vi "LSCI332 GetCtrlMode.vi"(0 "VISA Rsrc":refnum<visa-resource-name>="GPIB0::12::INSTR", 5 "Boucle(1)":u32(ring) caption="Boucle" items=["Boucle 1", "Boucle 2"], 11 "error in (no error)":errorcluster) -> (4 "Mode":u32(ring)=1 items=["Manual PID"=1, "Zone"=2, "Open Loop"=3, "AutoTune PID"=4, "AutoTune PI"=5, "AutoTune P"=6], 15 "error out":errorcluster)   [LabVIEW 2019]
doc: "Ce VI lit les paramètres limites de contrôle et ceux de stabilisation du contrôleur."
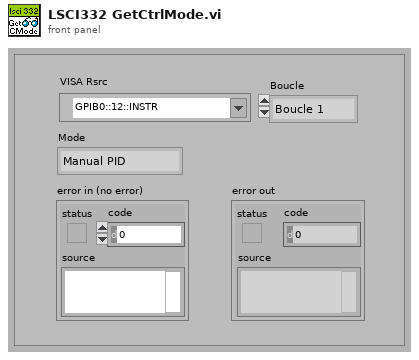
[diagram p1: front panel]
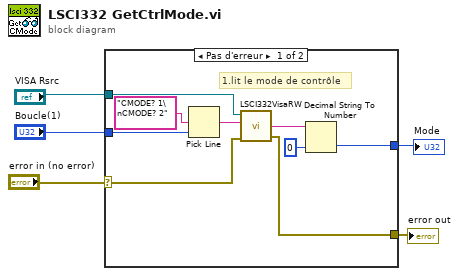
[diagram p0: block diagram]
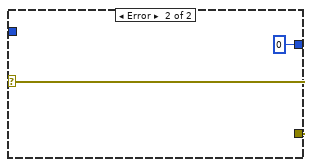
[diagram p2: hidden frame]
diagram:
  n1 = case shown="Pas d'erreur" "error in (no error)" {
    selector: "error in (no error)" -> [w13 w16]
    tunnel: "VISA Rsrc" -> [w14 _]
    tunnel: "Boucle(1)" -> [w11 _]
    tunnel: [w6 w16] -> w3
    tunnel: [w7 u32 0] -> w1
    frame No Error {
      # "1.lit le mode de contrôle"
      n2 = Pick Line(multi-line string="CMODE? 1\nCMODE? 2", line index=w11) -> (output string=w10:string)  [unwired: 1 in]
      n3 = call <userlib>:"LSCI332VisaRW.vi"("error in (no error)"=w13, "ChaineCom"=w10, "VISA Rsrc"=w14) -> ("error out"=w6:errorcluster, "ChaineRep"=w9:string)  [unwired: 4 in, 2 out]
      n4 = Decimal String To Number(string=w9, default (0L)=u32 0 ("default (0 I32)")) -> (number=w7:u32)  [unwired: 1 in, 1 out]
    }
    frame Error {
    }
  }
  "error out" <- w3
  "Mode" <- w1
